vi "Continuous Acquisition Off.vi"(8 "error in":errorcluster, 11 "Arduino Resource":T1={"VISA resource"="", "Board Type"=enum."Uno", "Connection Type"=enum."USB / Serial", "Bytes Per Packet (15)"=15}) -> (0 "error out":errorcluster, 3 "Arduino Resource":T1={"VISA resource"="", "Board Type"=enum."Uno", "Connection Type"=enum."USB / Serial", "Bytes Per Packet (15)"=15})   [LabVIEW 2015, in "LabVIEW Interface for Arduino.lvlib"]
doc: "This VI turns off continuous acquisition mode on the Arduino. After this VI is executed other Arduino function calls can be used again."
uses:
  <vilib>/LabVIEW Interface for Arduino/LabVIEW Interface for Arduino.lvlib
  <vilib>/LabVIEW Interface for Arduino/Type Defs/Arduino Resource.ctl
  <vilib>/LabVIEW Interface for Arduino/Type Defs/Board Type.ctl
  <vilib>/LabVIEW Interface for Arduino/Type Defs/Command.ctl
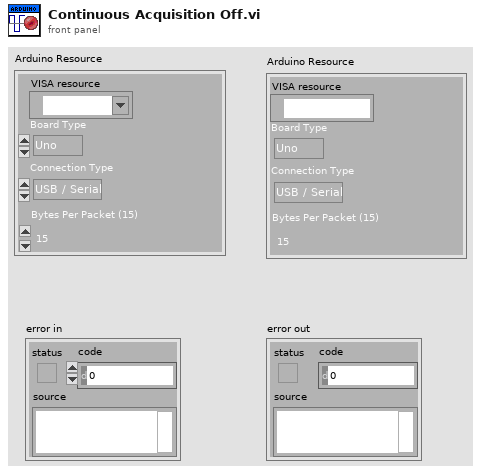
[diagram p1: front panel]
types:
  T1 = typedef "LabVIEW Interface for Arduino.lvlib/Arduino Resource.ctl" = cluster{"VISA resource":refnum<visa-resource-name>, "Board Type":T2, "Connection Type":enum8{"USB / Serial"}, "Bytes Per Packet (15)":u8}
  T2 = typedef "LabVIEW Interface for Arduino.lvlib/Board Type.ctl" = enum16{"Uno", "Dimuelanove w/Atmega 328", "Mega 2560"}
  T3 = typedef "LabVIEW Interface for Arduino.lvlib/Command.ctl" = enum8{"setArduinoMode", "flushSerial", "setPinMode", "digitalWritePin", "digitalWritePort", "tone", "digitalReadPin", "digitalReadPort", "analogReadPin", "analogReadPort", "pwmWritePin", "pwmWritePort", "sevenSegment_Configure", "sevenSegment_Write", "I2C Init", "I2C Write", "I2C Read", "SPI Init", "SPI Set Bit Order", "SPI Set Clock Divider", "SPI Set Data Mode", "SPI Send / Receive", "SPI Close", "Servo Set Num Servos", "Servo Config Servo", "Servo Write Angle", "Servo Read Angle", "Servo Write Pulse Width", "Servo Read Pulse Width", "Servo Detach", "LCD Init", "LCD Set Size", "LCD Set Cursor Mode", "LCD Clear", "LCD Set Cursor Position", "LCD Print", "LCD Display Power", "LCD Scroll Display", "LCD Autoscroll", "LCD Print Direction", "LCD Create Custom Char", "LCD Print Custom Char", "contAcqOn", "contAcqOff", "getFirmwareVersion", "FiniteSampleStart"}
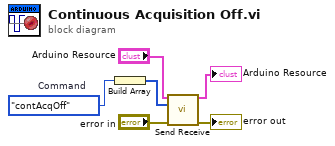
[diagram p0: block diagram]
diagram:
  w6 = Command."contAcqOff"  # Command
  n1 = Build Array(w6) -> (w5:T3[])
  n2 = call <vilib>:"Send Receive.vi"("Arduino Resource"="Arduino Resource", "Data"=w5, "error in"="error in") -> ("Arduino Resource"=→"Arduino Resource":T1, "error out"=→"error out":errorcluster)  [unwired: 10 in, 1 out]
